vi "DeployTest.vi"() -> ()   [LabVIEW 2016]
panel:
  out "Control Value:Get All":cluster{"Name":string, "Variant Data":variant}[](array[cluster])
  out "error out":errorcluster
  in  "Stop":bool
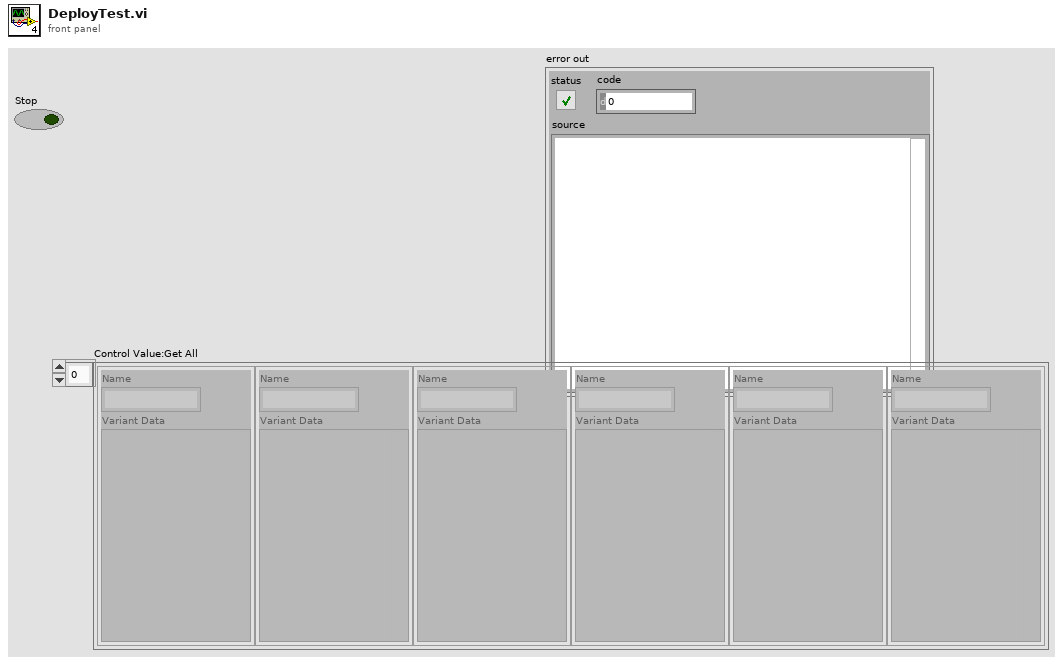
[diagram p1: front panel]
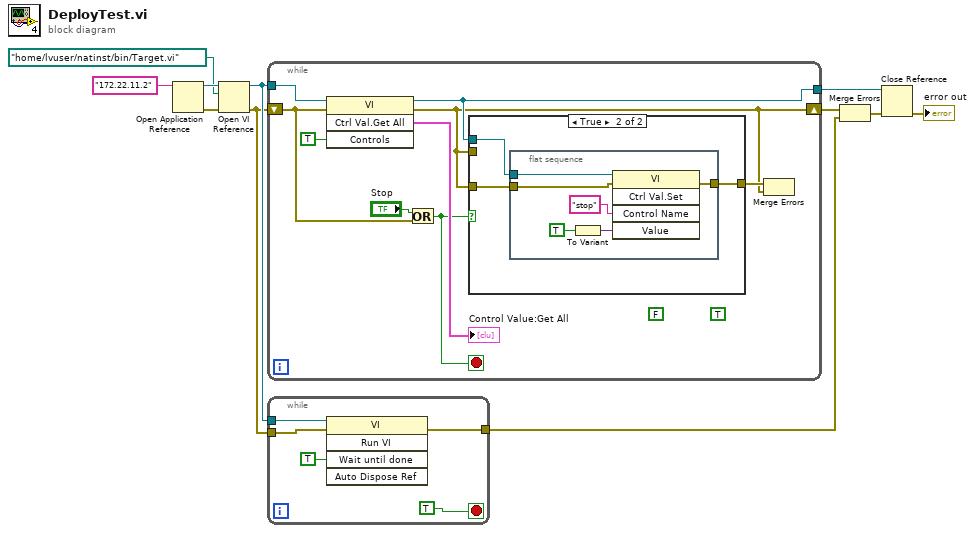
[diagram p0: block diagram]
diagram:
  n1 = Open Application Reference(11:"172.22.11.2" ("machine name (\"\":  open local reference)")) -> (0:w8:errorcluster, 3:w10:refnum<vi>)  [unwired: 3 in]
  n2 = Open VI Reference(application reference (local)=w10, vi path=path "/home/lvuser/natinst/bin/Target.vi", error in (no error)=w8) -> (vi reference=w6:refnum<vi>, error out=w4:errorcluster)  [unwired: 3 in]
  n3 = while {
    shift-right: [w13] -> w3
    shift-left: w4 -> [w20]
    tunnel: [w15] -> w7
    tunnel: w6 -> [w17]
    stop <- w12 stop-if-true
    (unwired) TRUE ("Wait Until Done")
    (unwired) FALSE ("Wait Until Done")
    n4 = invoke class="VI" method="Ctrl Val.Get All"(reference=w17, error in=w20, "Controls"=TRUE) -> (reference out=w15:refnum<vi>, error out=w13:errorcluster, "Get All Control Values Variant"=→"Control Value:Get All":cluster{"Name":string, "Variant Data":variant}[])  [unwired: 1 in, 1 out]
    n5 = Or(x="Stop", y=w20) -> (x .or. y?=w12:bool)
    n6 = case shown="True" w12 {
      tunnel: w15 -> [_ w24]
      tunnel: [w21 w23] -> w14
      tunnel: w13 -> [w21 _]
      tunnel: w13 -> [_ w22]
      frame False {
      }
      frame True {
        n7 = flat-sequence {
          tunnel: w24 -> [w29]
          tunnel: [w28] -> w23
          tunnel: w22 -> [w27]
          frame #0 {
            n8 = To Variant(anything=TRUE ("Stop")) -> (Variant=w26:variant)
            n9 = invoke class="VI" method="Ctrl Val.Set"(reference=w29, error in=w27, "Control Name"="stop", "Value"=w26) -> (error out=w28:errorcluster)  [unwired: 1 in, 4 out]
          }
        }
      }
    }
    n10 = Merge Errors(w14, w13) -> ()  [unwired: 1 out]
  }
  n11 = while {
    tunnel: w6 -> [w35]
    tunnel: [w33] -> w5
    tunnel: w4 -> [w32]
    stop <- TRUE stop-if-true
    n12 = invoke class="VI" method="Run VI"(reference=w35, error in=w32, "Wait until done"=TRUE ("Wait Until Done")) -> (error out=w33:errorcluster)  [unwired: 2 in, 4 out]
  }
  n13 = Merge Errors(w3, w5) -> (w2:errorcluster)
  n14 = Close Reference(reference=w7, error in (no error)=w2) -> (error out=→"error out":errorcluster)
